vi "PicoScope2000aSetEtsTimeBuffer.vi"(8 "error in (no error)":errorcluster, 10 "bufferLth":i32, 11 "handle in":i16) -> (0 "error out":errorcluster, 2 "EtsTimeValues":i64[](array[numeric]), 3 "handle out":i16)   [LabVIEW 2010]
doc: "Calls SetEtsTimeBuffer"
uses:
  ps2000a.dll
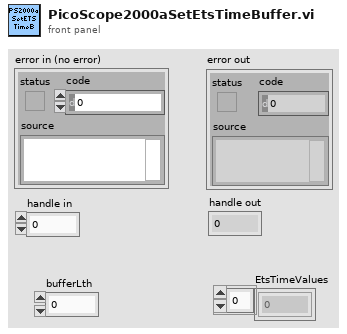
[diagram p1: front panel]
types:
  T1 = enum16{"U8", "I8", "U16", "I16", "U32", "I32", "U64", "I64"}
  T2 = cluster{"status":bool, "code":u32, "source":string}
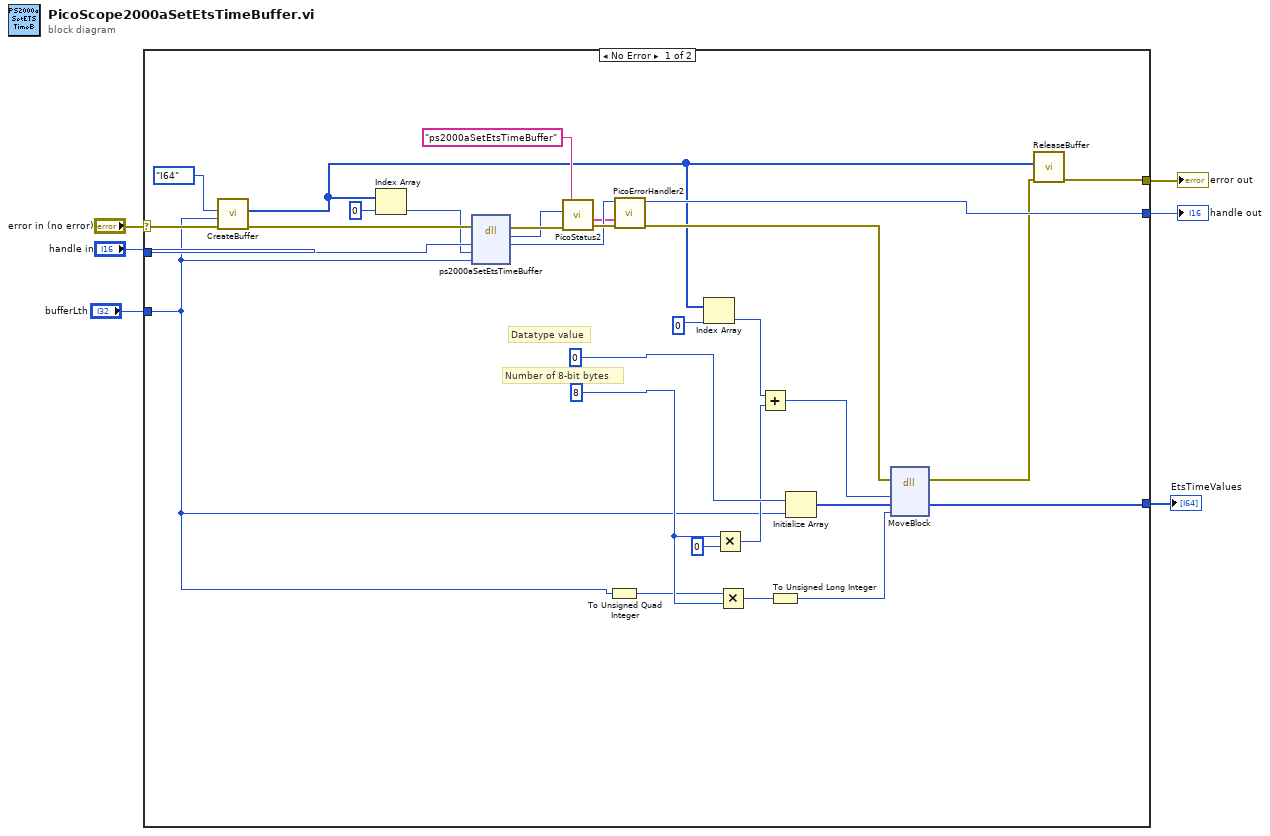
[diagram p0: block diagram]
diagram:
  n1 = case shown="No Error" "error in (no error)" {
    selector: "error in (no error)" -> [w29 w37]
    tunnel: [w27 w37] -> w4
    tunnel: "handle in" -> [w33 w36]
    tunnel: [w30 w36] -> w5
    tunnel: "bufferLth" -> [w8 _]
    tunnel: [w13 _] -> w1
    frame No Error {
      w21 = u64 8 ("y")
      # "Number of 8-bit bytes"
      # "Datatype value"
      n2 = call "CreateBuffer.vi"("error in (no error)"=w29, "Buffer size"=w8, "Data type"=T1."I64") -> ("error out"=w28:errorcluster, "Pointer and BufferSize"=w11:u64[])  [unwired: 7 in]
      n3 = Index Array(array=w11, index=0) -> (element=w26:u64)
      n4 = dll-call lib="ps2000a.dll" fn="ps2000aSetEtsTimeBuffer" ("ps3000.dll:_ps3000_open_unit@0")(error in=w28, "handle"=w33, "buffer"=w26, "bufferLth"=w8) -> (error out=w32:errorcluster, "PICO_STATUS"=w31:u32, "handle"=w30:i16)  [unwired: 4 in, 1 out]
      n5 = call "PicoStatus2.vi"("PICO source"="ps2000aSetEtsTimeBuffer" ("source"), "Error in"=w32, "PICO STATUS"=w31) -> ("error out"=w35:errorcluster, "PICO_STATUS out"=w7:T2)  [unwired: 5 in]
      n6 = To Unsigned Quad Integer(1:w8) -> (0:w9:u64)
      n7 = call "PicoErrorHandler2.vi"("error in (no error)"=w35, "PICO_STATUS in"=w7, "handle In"=w30) -> ("error out"=w14:errorcluster)  [unwired: 8 in]
      n8 = Index Array(array=w11, index=0) -> (element=w23:u64)
      n9 = Multiply(x=w21, y=u64 0) -> (x*y=w22:u64)
      n10 = Multiply(x=w9, y=w21) -> (x*y=w20:u64)
      n11 = Add(x=w23, y=w22) -> (x+y=w19:u64)
      n12 = To Unsigned Long Integer(number=w20) -> (unsigned 32bit integer=w17:u32)
      n13 = Initialize Array(i64 0 ("element"), w8) -> (w18:i64[])
      n14 = dll-call lib="LabVIEW" fn="MoveBlock"(error in=w14, "Source"=w19, "Destination"=w18, "Size"=w17) -> (error out=w15:errorcluster, "Destination"=w13:i64[])  [unwired: 5 in, 1 out]
      n15 = call "ReleaseBuffer.vi"("error in (no error)"=w15, "Pointer and BufferSize"=w11) -> ("error out"=w27:errorcluster)  [unwired: 9 in]
    }
    frame Error {
    }
  }
  "error out" <- w4
  "handle out" <- w5
  "EtsTimeValues" <- w1
